vi "queMN.vi"(8 "error in (no error)":errorcluster caption="错误输入（无错误）", 10 "簇":cluster{"MN":string, "PW":string}={"MN"="平台数据发送系统", "PW"="平台数据发送系统"}, 11 "interface 输入":refnum<class "interface.lvclass">) -> (0 "error out":errorcluster caption="错误输出", 2 "包含启动项":bool, 3 "interface 输出":refnum<class "interface.lvclass">)   [LabVIEW 2016, in "interface.lvclass"]
uses:
  interface.lvclass
  <vilib>/registry/registry.llb/Registry RtKey.ctl
  <vilib>/registry/registry.llb/Read Registry Value Simple STR.vi
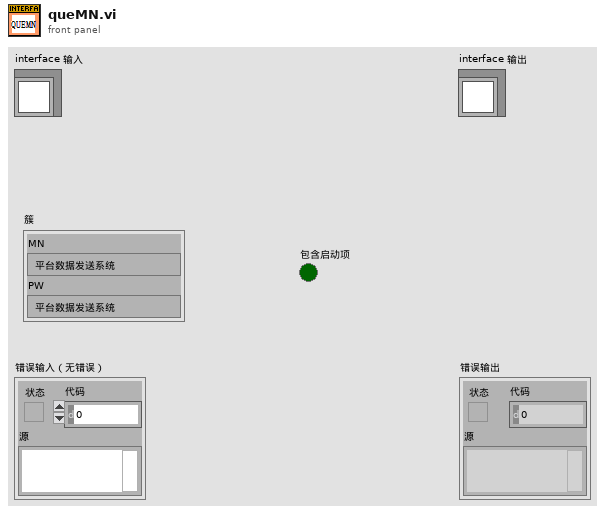
[diagram p1: front panel]
types:
  T1 = typedef "Registry RtKey.ctl" = enum32{"HKEY_CLASSES_ROOT", "HKEY_CURRENT_USER", "HKEY_LOCAL_MACHINE", "HKEY_USERS", "HKEY_PERFORMANCE_DATA", "HKEY_CURRENT_CONFIG", "HKEY_DYN_DATA"}
  T2 = typedef "Registry refnum.ctl" = refnum<k1>
  T3 = cluster{"numValues":i32, "maxValueNameLen":i32, "maxValueDataLen":i32}
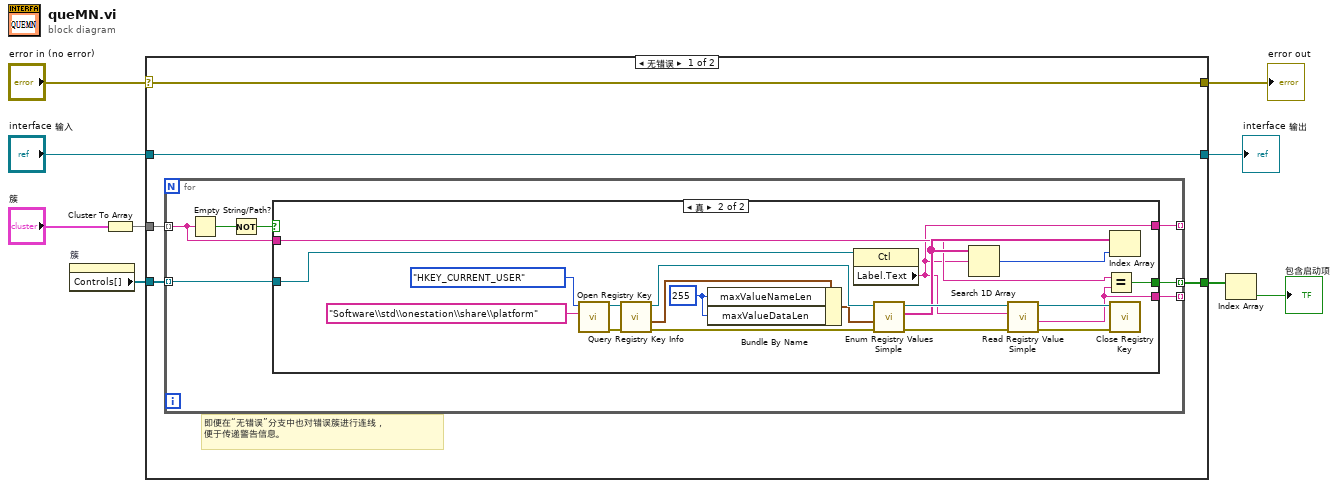
[diagram p0: block diagram]
diagram:
  n1 = property on="簇" class="Clust (严格)"() -> ("Controls[]"=w2:refnum<vi>[])  [unwired: 2 in, 2 out]
  n2 = Cluster To Array(cluster="簇") -> (array=w3:string[])
  n3 = case shown="无错误" "error in (no error)" {
    selector: "error in (no error)" -> [w13 w43]
    tunnel: [w13 w43] -> w8
    tunnel: [w14 w42] -> w6
    tunnel: "interface 输入" -> [w14 w42]
    tunnel: w3 -> [w12 _]
    tunnel: w2 -> [w11 _]
    tunnel: [w10 _] -> w1
    frame No Error {
      # "即便在“无错误”分支中也对错误簇进行连线，\n便于传递警告信息。"
      n4 = for {
        tunnel: w12 -> [w19] mode=indexing
        tunnel: w11 -> [w18] mode=indexing
        tunnel: [w17] -> _ mode=indexing
        tunnel: [w16] -> w10 mode=indexing
        tunnel: [w15] -> _ mode=indexing
        n5 = Empty String/Path?(string/path=w19) -> (empty?=w21:bool)
        n6 = Not(x=w21) -> (.not. x?=w20:bool)
        n7 = case shown="真" w20 {
          tunnel: [_ w30] -> w16
          tunnel: w19 -> [_ w23]
          tunnel: w18 -> [_ w26]
          tunnel: [_ w25] -> w17
          tunnel: [_ w22] -> w15
          frame False {
          }
          frame True {
            w27 = 255 ("maxValueNameLen")
            n8 = call <vilib>:"Open Registry Key.vi"("subkey"="Software\\std\\onestation\\share\\platform", "root key (HKEY_LOCAL_MACHINE)"=Registry_RtKey."HKEY_CURRENT_USER") -> ("error out"=w38:errorcluster, "refnum out"=w39:T2)  [unwired: 8 in]
            n9 = call <vilib>:"Query Registry Key Info.vi"("error in (no error)"=w38, "refnum"=w39) -> ("error out"=w36:errorcluster, "value info"=w29:T3, "refnum out"=w37:T2)  [unwired: 5 in, 2 out]
            n10 = Bundle By Name(cluster=w29, "maxValueNameLen"=w27, "maxValueDataLen"=w27) -> (w28:T3)
            n11 = property class="Ctl"(reference=w26) -> ("Label.Text"=w22:string)  [unwired: 1 in, 2 out]
            n12 = call <vilib>:"Enum Registry Values Simple.vi"("error in (no error)"=w36, "value info"=w28, "refnum"=w37) -> ("error out"=w33:errorcluster, "values"=w24:string[], "refnum out"=w35:T2)  [unwired: 3 in, 3 out]
            n13 = Search 1D Array(1D array=w24, element=w22) -> (index of element=w31:i32)  [unwired: 1 in]
            n14 = call-poly <vilib>:"Read Registry Value Simple.vi"("error in (no error)"=w33, "value"=w22, "refnum"=w35) -> ("error out"=w32:errorcluster, "String/Binary data"=w25:string, "refnum out"=w34:T2)  [unwired: 3 in, 1 out]
            n15 = Equal?(x=w23, y=w25) -> (x = y?=w30:bool)
            n16 = Index Array(array=w24, index=w31) -> ()  [unwired: 1 out]
            n17 = call <vilib>:"Close Registry Key.vi"("error in (no error)"=w32, "refnum"=w34) -> ()  [unwired: 5 in, 1 out]
          }
        }
      }
    }
    frame Error {
    }
  }
  "error out" <- w8
  "interface 输出" <- w6
  n18 = Index Array(array=w1) -> (element=→"包含启动项":bool)  [unwired: 1 in]
